vi "FSA.vi"(0 "System no.":i32=1 min=1 step=1, 1 "Board":i32=1 min=1 max=5 step=1, 2 "Axis 1 to scan":string, 3 "Axis 2 to scan":string, 4 "Range axis 1":dbl=0.1 format="%.4f", 5 "error in":errorcluster, 6 "Treshold level":dbl=0.1 format="%.3f", 7 "Step size":dbl=0.05 format="%.4f", 8 "AA Step size":dbl=0.05 format="%.4f", 9 "Range axis 2":dbl=0.1 format="%.4f", 10 "Use #7 polling?":bool, 11 "Timeout (s)":dbl=300.0 min=1.0 max=4.0 step=1.0 format="%.2f", 12 "Stop refnum":refnum<vi>) -> (14 "Scan successful?":bool, 19 "error out":errorcluster)   [LabVIEW 2026]
doc: "Performs a 2D scan and align in specified axes, waits until scan is ready using #7 polling (if checked) and indicates whether scan was successful or not. If Stop refnum or Local stop is TRUE, VI sends #24 and stops. For a square scan, Range axis 2 must be identical to Range axis 1, otherwise a rectangular scan is performed. Timeout is only valid if Use #7 polling is FALSE.\n\nC-880: Use #7 polling = TRUE\nC-887, F-206, M-8X0: Use #7 polling = FALSE, Range axis 2 must be identical with Range axis 1 (no rectangular scan implemented). For GCS syntax version = GCS 2.0 or higher (check with CSV?.vi. If CSV?.vi is not supported, syntax version is GCS 1.0), VI calls FSS? automatically to determine if scan was successful or not."
uses:
  Communication/Syntax.ctl
  Communication/Global1.vi
panel:
  in  "Local stop":bool
  # "Performs an 2D scan and align in specified axes, waits until scan is ready (using \n#7 polling if checked) and indicates whether scan was successful or not.  If Stop \nrefnum or Local stop is TRUE, VI sends #24 and stops. For a square scan, \"Range \naxis 2\" must be identical to \"Range axis 1\", otherwise a rectangular scan is \nperformed. \"Timeout\" is only valid if \"Use #7 polling\" is FALSE."
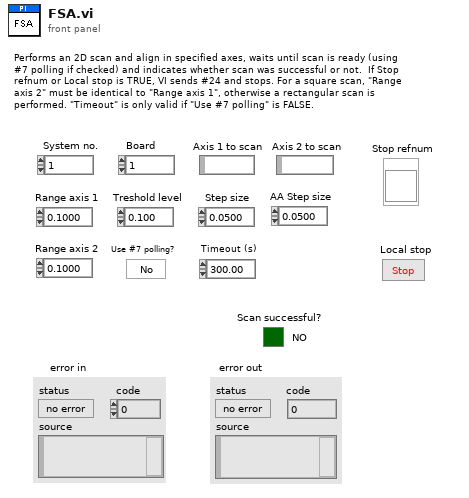
[diagram p1: front panel]
types:
  T1 = typedef "Syntax.ctl" = enum16{"GCS 1.0", "GCS 2.0", "GCS 3.0"}
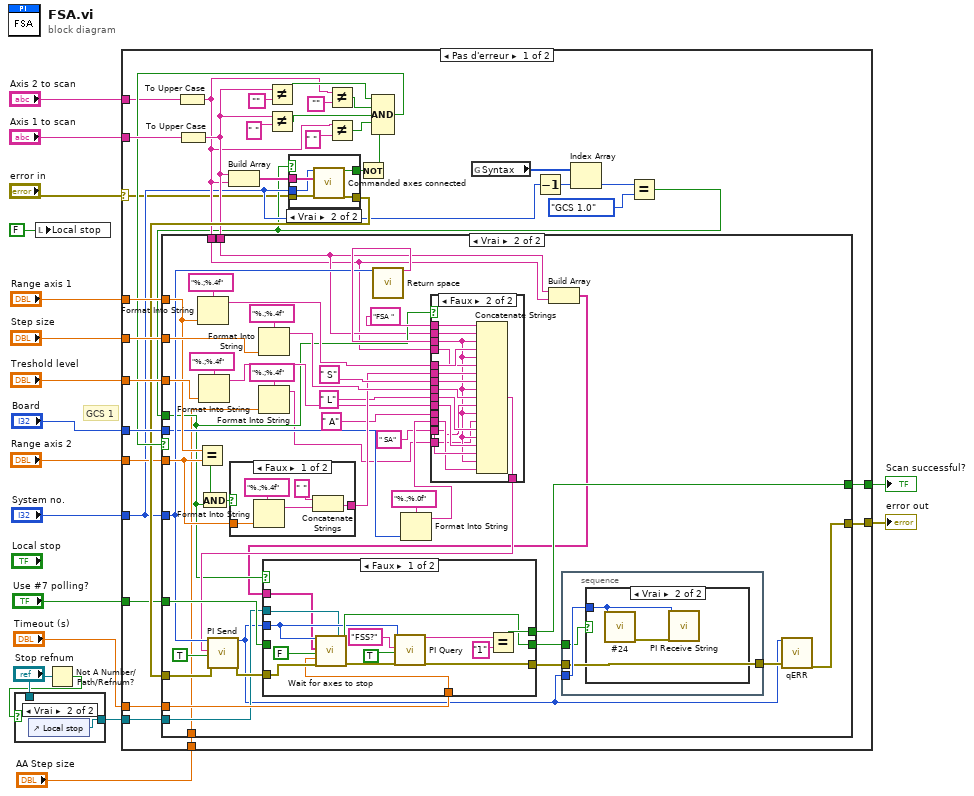
[diagram p0: block diagram]
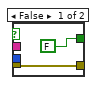
[diagram p3: hidden frame]
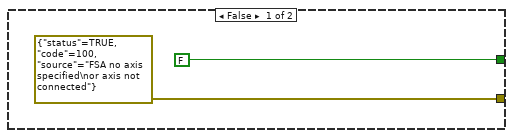
[diagram p4: hidden frame]
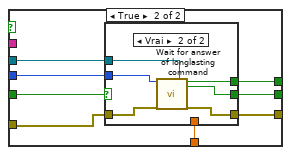
[diagram p5: hidden frame]
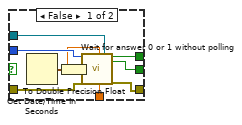
[diagram p6: hidden frame]
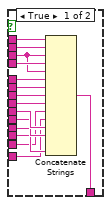
[diagram p7: hidden frame]
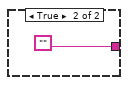
[diagram p9: hidden frame]
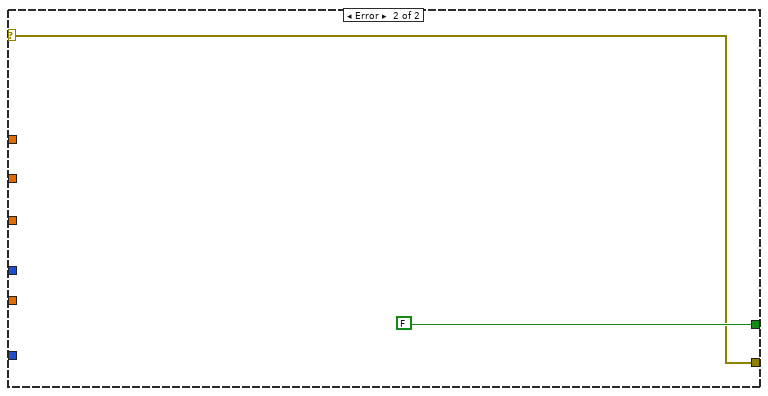
[diagram p10: hidden frame]
diagram:
  # "GCS 1"
  n1 = local write "Local stop"(FALSE ("Local stop")) -> ()
  n2 = Not A Number/Path/Refnum?(number/path/refnum="Stop refnum") -> (NaN/Path/Refnum?=w4:bool)
  n3 = case shown="Vrai" w4 {
    tunnel: [w19 w20] -> w3
    tunnel: "Stop refnum" -> [w19 _]
    frame False {
    }
    frame True {
      n4 = control-ref of="Local stop"() -> (w20:refnum<vi>)
    }
  }
  n5 = case shown="Pas d'erreur" "error in" {
    selector: "error in" -> [w22 w185]
    tunnel: "System no." -> [w25 _]
    tunnel: [w44 w185] -> w17
    tunnel: "Axis 1 to scan" -> [w55 _]
    tunnel: [w43 FALSE] -> w15
    tunnel: "Board" -> [w50 _]
    tunnel: "Range axis 1" -> [w49 _]
    tunnel: "Step size" -> [w48 _]
    tunnel: "Treshold level" -> [w47 _]
    tunnel: "Axis 2 to scan" -> [w39 _]
    tunnel: "Use #7 polling?" -> [w32 _]
    tunnel: "Timeout (s)" -> [w31 _]
    tunnel: "Range axis 2" -> [w30 _]
    tunnel: w3 -> [w29 _]
    tunnel: "AA Step size" -> [w23 _]
    frame No Error {
      n6 = To Upper Case(1:w39) -> (0:w33:string)
      n7 = To Upper Case(1:w55) -> (0:w34:string)
      n8 = Build Array(w34, w33) -> (w51:string[])
      n9 = Not Equal?(x=w34, y="") -> (x != y?=w52:bool)
      n10 = Not Equal?(x=w34, y=" ") -> (x != y?=w37:bool)
      n11 = Not Equal?(x=w33, y="") -> (x != y?=w36:bool)
      n12 = Not Equal?(x=w33, y=" ") -> (x != y?=w35:bool)
      n13 = global read "Global1.vi" "Syntax"() -> (w26:T1[])
      n14 = Decrement(x=w25) -> (x-1=w27:i32)
      n15 = Index Array(array=w26, index=w27) -> (element=w28:T1)
      n16 = Equal?(x=w28, y=Syntax."GCS 1.0") -> (x = y?=w24:bool)
      n17 = case shown="Vrai" w24 {
        tunnel: w51 -> [_ w62]
        tunnel: w22 -> [w56 w61]
        tunnel: [w56 w60] -> w45
        tunnel: [FALSE ("Controller error") w59] -> w42
        tunnel: w25 -> [_ w58]
        frame False {
        }
        frame True {
          n18 = call "Commanded axes connected.vi"("System no."=w58, "Commanded axes"=w62, "error in"=w61) -> ("Controller error"=w59:bool, "error out"=w60:errorcluster)  [unwired: 15 out]
        }
      }
      n19 = Not(x=w42) -> (.not. x?=w41:bool)
      n20 = Compound Arithmetic op=AND(w52, w36, w37, w35, w41) -> (w46:bool)
      n21 = case shown="Vrai" w46 {
        tunnel: w50 -> [_ w75]
        tunnel: w49 -> [_ w93]
        tunnel: w48 -> [_ w99]
        tunnel: w34 -> [_ w71]
        tunnel: w47 -> [_ w101]
        tunnel: w45 -> [_ w106]
        tunnel: w25 -> [_ w80]
        tunnel: [errorcluster {"status"=TRUE, "code"=100, "source"="FSA no axis specified\nor axis not connected"} ("error out") w87] -> w44
        tunnel: [FALSE w86] -> w43
        tunnel: w33 -> [_ w70]
        tunnel: w32 -> [_ w97]
        tunnel: w31 -> [_ w96]
        tunnel: w30 -> [_ w92]
        tunnel: w29 -> [_ w83]
        tunnel: w24 -> [_ w72]
        tunnel: w23 -> [_ w66]
        frame False {
        }
        frame True {
          n22 = Equal?(x=w93, y=w92) -> (x = y?=w79:bool)
          n23 = Format Into String(format string="%.;%.4f" ("Format String"), w93) -> (resulting string=w98:string)  [unwired: 2 in, 1 out]
          n24 = Format Into String(format string="%.;%.4f" ("Format String"), w101) -> (resulting string=w89:string)  [unwired: 2 in, 1 out]
          n25 = And(x=w79, y=w72) -> (x .and. y?=w78:bool)
          n26 = case shown="Faux" w78 {
            tunnel: w92 -> [w182 _]
            tunnel: [w179 ""] -> w91
            frame False {
              n27 = Format Into String(format string="%.;%.4f" ("Format String"), w182) -> (resulting string=w180:string)  [unwired: 2 in, 1 out]
              n28 = Concatenate Strings(" ", w180) -> (w179:string)
            }
            frame True {
            }
          }
          n29 = Format Into String(format string="%.;%.4f" ("Format String"), w99) -> (resulting string=w95:string)  [unwired: 2 in, 1 out]
          n30 = Format Into String(format string="%.;%.4f" ("Format String"), w66) -> (resulting string=w65:string)  [unwired: 2 in, 1 out]
          n31 = call "Return space.vi"("System no."=w80) -> ("String out"=w81:string)  [unwired: 1 in, 17 out]
          n32 = Format Into String(format string="%.;%.0f" ("Format String"), w75) -> (resulting string=w74:string)  [unwired: 2 in, 1 out]
          n33 = case shown="Faux" w72 {
            tunnel: [w158 w173] -> w73
            tunnel: w98 -> [w157 w166]
            tunnel: w95 -> [w156 w172]
            tunnel: " S" -> [w155 w171]
            tunnel: w91 -> [w154 w164]
            tunnel: " L" -> [w153 w170]
            tunnel: w89 -> [w152 w169]
            tunnel: "FSA " -> [w151 w168]
            tunnel: w71 -> [w150 w167]
            tunnel: w70 -> [w149 w165]
            tunnel: w81 -> [w148 w160]
            tunnel: " A" -> [w147 w163]
            tunnel: w74 -> [w146 w162]
            tunnel: " SA" -> [w145 w161]
            tunnel: w65 -> [w144 w159]
            frame True {
              n34 = Concatenate Strings(w151, w150, w148, w149, w148, w157, w154, w155, w156, w145, w144, w153, w152, w147, w146) -> (w158:string)
            }
            frame False {
              n35 = Concatenate Strings(w168, w167, w160, w166, w160, w165, w164, w171, w160, w172, w161, w160, w159, w170, w160, w169, w163, w160, w162) -> (w173:string)
            }
          }
          n36 = call "PI Send.vi"("System no."=w80, "String to send"=w73, "Attach termination char.?"=TRUE ("Attach Linefeed?"), "error in"=w106) -> ("error out"=w104:errorcluster)  [unwired: 2 in, 13 out]
          n37 = Build Array(w71, w70) -> (w69:string[])
          n38 = case shown="Faux" w72 {
            tunnel: w104 -> [w115 w128]
            tunnel: w97 -> [_ w127]
            tunnel: w96 -> [w110 w126]
            tunnel: [w114 w125] -> w86
            tunnel: [w108 w124] -> w85
            tunnel: [w113 w123] -> w84
            tunnel: w83 -> [w111 w122]
            tunnel: w80 -> [w112 w121]
            tunnel: w69 -> [w109 _]
            frame False {
              n39 = call "Wait for axes to stop.vi"("System no."=w112, "Axes to wait for"=w109, "With status bit polling?"=FALSE, "Timeout (s)"=w110, "error in"=w115, "Stop refnum"=w111) -> ("Stopped"=w113:bool, "error out"=w117:errorcluster)  [unwired: 1 in, 11 out]
              n40 = call "PI Query.vi"("System no."=w112, "String to send"="FSS?", "Attach termination char.?"=TRUE ("Attach Linefeed?"), "error in"=w117) -> ("String read"=w107:string, "error out"=w108:errorcluster)  [unwired: 3 in, 11 out]
              n41 = Equal?(x=w107, y="1") -> (x = y?=w114:bool)
            }
            frame True {
              n42 = case shown="Vrai" w127 {
                tunnel: w121 -> [w137 w143]
                tunnel: w128 -> [w136 w142]
                tunnel: [w135 w141] -> w124
                tunnel: [w134 w140] -> w125
                tunnel: w126 -> [w132 _]
                tunnel: [w130 w139] -> w123
                tunnel: w122 -> [w131 w138]
                frame False {
                  n43 = Get Date/Time In Seconds() -> (seconds since 1Jan1904=w129:timestamp)
                  n44 = To Double Precision Float(number=w129) -> (double precision float=w133:dbl)
                  n45 = call "Wait for answer 0 or 1 without polling.vi"("System no."=w137, "error in"=w136, "Start time"=w133, "Timeout (s)"=w132, "Stop refnum"=w131) -> ("Scan successful?"=w134:bool, "Stopped"=w130:bool, "error out"=w135:errorcluster)  [unwired: 12 out]
                }
                frame True {
                  n46 = call "Wait for answer of longlasting command.vi"("System no."=w143, "error in"=w142, "Stop refnum"=w138) -> ("Answer"=w140:bool, "Stopped"=w139:bool, "error out"=w141:errorcluster)  [unwired: 14 out]
                }
              }
            }
          }
          n47 = stacked-sequence {
            tunnel: w80 -> [w176]
            tunnel: w85 -> [w175]
            tunnel: [w175] -> w88
            tunnel: w84 -> [w174]
            frame #0 {
              n48 = case shown="Vrai" w174 {
                tunnel: w176 -> [_ w178]
                frame False {
                }
                frame True {
                  n49 = call "#24.vi"("System no."=w178) -> ("error out"=w177:errorcluster)  [unwired: 1 in, 17 out]
                  n50 = call "PI Receive String.vi"("System no."=w178, "error in"=w177) -> ()  [unwired: 1 in, 17 out]
                }
              }
            }
          }
          n51 = call "qERR.vi"("System no."=w80, "error in"=w88) -> ("error out"=w87:errorcluster)  [unwired: 17 out]
        }
      }
    }
    frame Error {
    }
  }
  "error out" <- w17
  "Scan successful?" <- w15
